vi "Lab8-PSK_Simulation_4PSK_Simple(1).vi"() -> ()   [LabVIEW 2013]
uses:
  <vilib>/addons/Modulation/Digital/General/MT Generate Bits (Galois, PN Order).vi
  <vilib>/addons/Modulation/Digital/General/MT Generate PSK System Parameters(M).vi
  <vilib>/addons/Modulation/Digital/General/MT Generate PSK Synchronization Parameters (bit array).vi
  <vilib>/addons/Modulation/Digital/General/MT Format Eye Diagram (complex).vi
  <vilib>/addons/Modulation/niDMT.lvlib
panel:
  out "sync found index (symbols)":dbl format="%.4f"
  in  "Eb/N0 (dB)":dbl(slide)=48.26086956521739 scale=-10.0..50.0
  out "measurements":T1 caption="Measurements" {"phase offset (deg)" format="%.2f"; "frequency drift (Hz)" format="%.2f"; "frequency offset (Hz)" format="%.2f"}
  out "Baseband Waveform":cluster{"t0":dbl, "dt":dbl, "Y":dbl[]}(graph)
  in  "Tab Control":enum32{"Constellation", "Eye Diagram"}(tab)
  out "Constellation Plot":T2(graph)=[{"constellation"=[-0.6843393450045908, -0.7188173867833647, -0.6862679721424542, -0.7297030487459608, -0.7159912856499204, 0.7221248350001428, -0.69319374455267, -0.7177933374862676, 0.6893145049073991, 0.7164949508669772, -0.7136233597527977, 0.7088022813066004, 0.7026806753460019, 0.6993908820448104, 0.7033303803758204, 0.7023239283689477, -0.7092821972958672, 0.7043694263023035, -0.71123073342578, -0.7063013580615412, 0.7025174893431778, -0.7079249457114573, 0.7056952690720733, -0.711060440916994, -0.7135916049305011, -0.7042966683375681, -0.7053639500078486, -0.7170793110386893, 0.7007122470722706, -0.7041907238690962, 0.7069307076270948, -0.7303032352912369, 0.7036742608538313, -0.7213763894899665, 0.6974920430188264, -0.6906276182534745, 0.7110338385529501, 0.707668395707459, 0.7066450908567875, 0.7156573983712801, 0.7058430026446071, 0.7226424194495579, -0.6941394170921843, 0.7153952742388731, -0.7061754291757949, 0.6989077999376425, 0.7322949703863137, -0.7277124364880128, 0.7152053555332901, -0.7144386806873485, 0.7122523333502172, -0.6946532350705298, -0.6977995339788963], "oversampled data"=[-0.6885507056398621, -0.6904021301332153, -0.701720009748651, 0.7230147663617461, 0.6792985003415442, 0.714980330495899, 0.7083798924531897, -0.7030264642885489, 0.7016069656212314, -0.6995735246622811, -0.7187083014951974, 0.718556461974981, -0.7154964369422703, -0.7143626925937305, -0.7168215682367294, 0.6901290658424636, 0.7193430662186729, 0.7021618219264352, -0.7044915371643418, 0.7010427354068245, 0.72862911894502, -0.6931780204687834, -0.7208414620302925, 0.6898461638663613, 0.7171050214665211, 0.7071101521691305, -0.7158811583840712, 0.7100771986297291, 0.7055043383295747, 0.7197934468495215, -0.7126751015343431, 0.699715799910657, 0.7071055136917425, 0.7000396806158872, 0.6959369636505729, 0.7171363071737368, 0.7097950846368283, 0.707670861017943, 0.6989567675175453, -0.7157042609479739, 0.7040676123623458, 0.7131191099779645, 0.7010491472655718, 0.7001052143691281, -0.7044803945850813, 0.6953086657664377, 0.7183481414573912, 0.7015721146800344, -0.6848840235343148, -0.712341720231345, 0.7005395668208682, 0.6964886799304421, 0.6911618122252481]}, {"constellation"=array[848 elements], "oversampled data"=array[848 elements]}]
  out "Eye Diagram":cluster{"t0":dbl, "dt":dbl, "Y":dbl[]}[](graph)
  in  "M-PSK (4)":i32=4
  out "LED Array":T3
  in  "Message Bits":i32=100
  out "error out":errorcluster
  in  "stop 2":bool
  # "M-PSK Simulation"
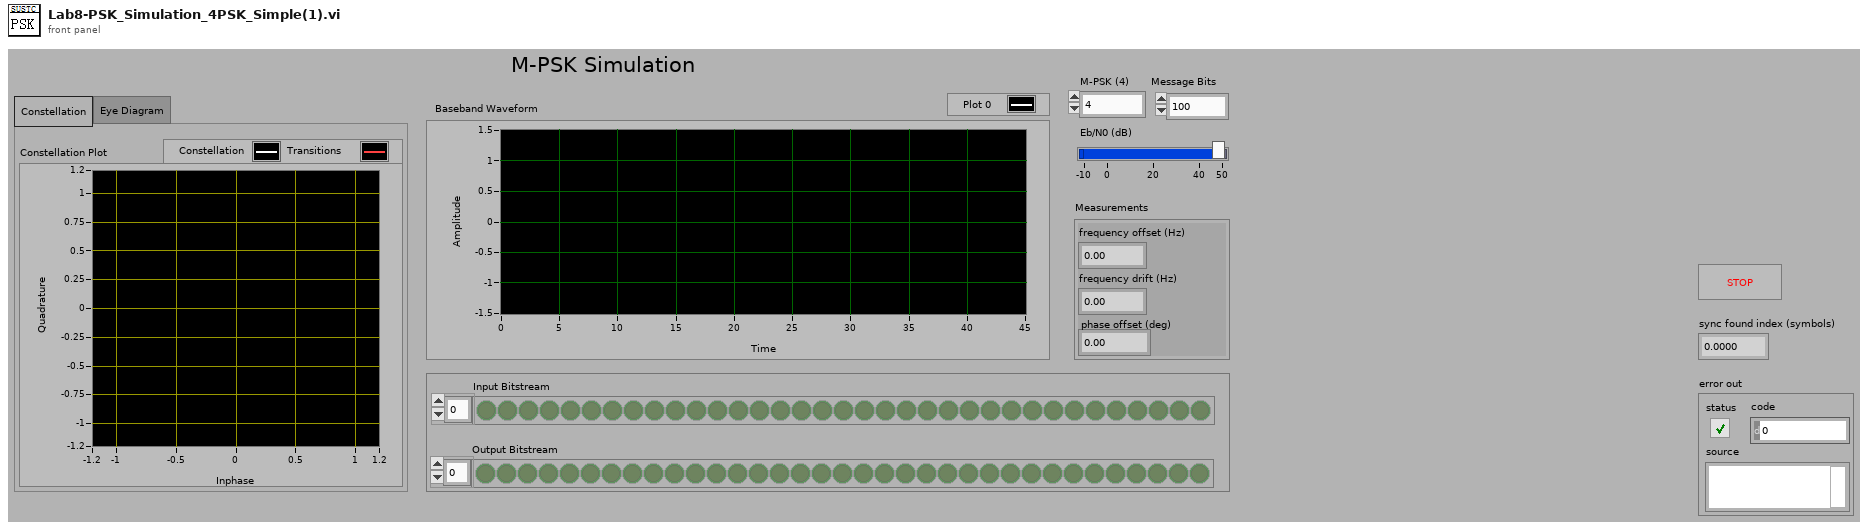
[diagram p1: front panel]
types:
  T1 = cluster{"frequency offset (Hz)":dbl, "frequency drift (Hz)":dbl, "phase offset (deg)":dbl}
  T2 = cluster{"constellation":dbl[], "oversampled data":dbl[]}[]
  T3 = cluster{"Input Bitstream":bool[], "Output Bitstream":bool[]}
  T4 = enum16{"none", "Raised Cosine", "Root Raised Cos", "Gaussian"}
  T5 = enum16{"FSK", "PSK", "QAM", "MSK", "PAM", "ASK", "CPM"}
  T6 = cluster{"samples per symbol (16)":i32, "symbol map":cdb[], "differential PSK":enum16{"disable", "enable"}, "PSK type":u16}
  T7 = typedef "niAMT.lvlib/Complex Data Waveform.ctl" = cluster{"t0":dbl, "dt":dbl, "Y":cdb[]}
  T8 = cluster{"expected sync location (symbols)":i32, "sync sequence":cdb[], "sync location uncertainty (symbols)":i32, "sync indent (symbols)":i32}
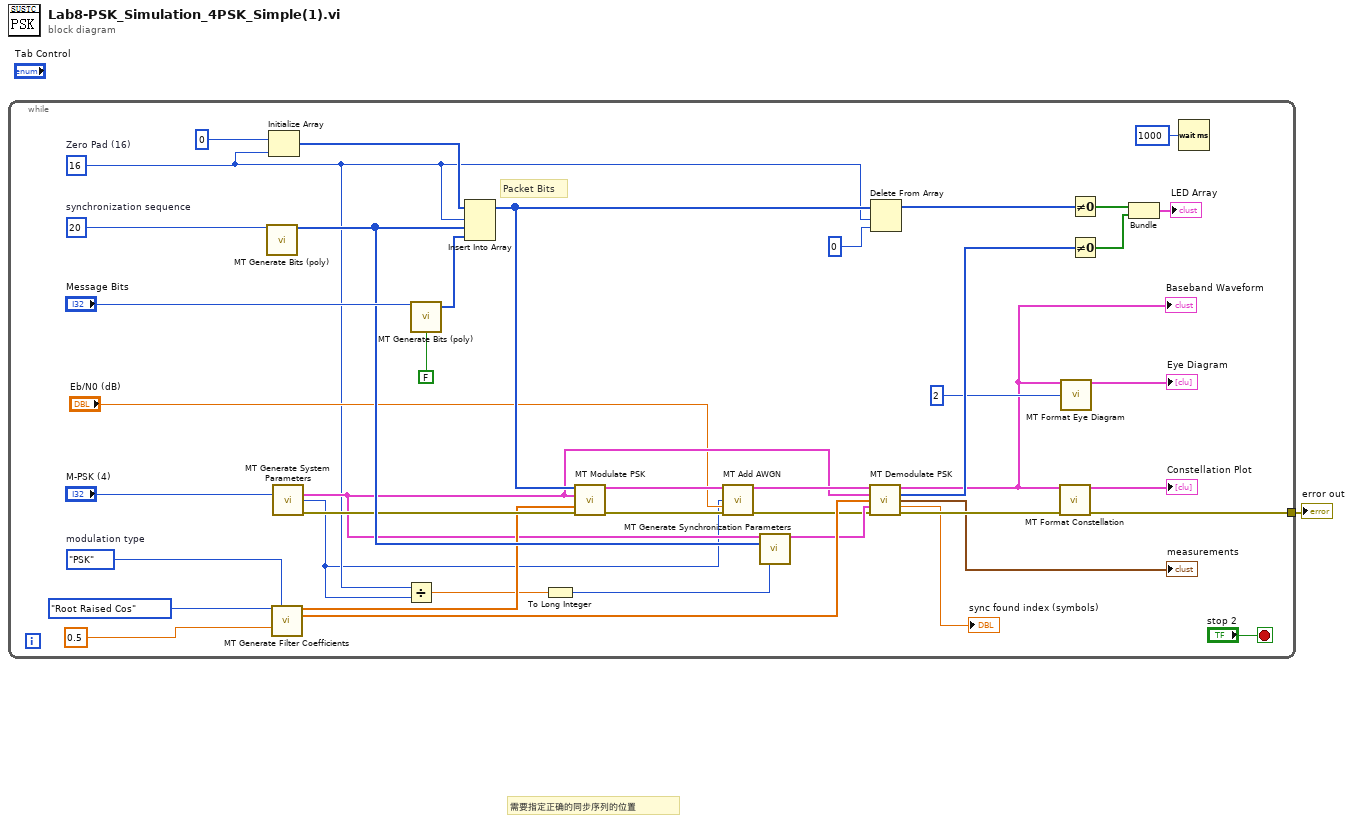
[diagram p0: block diagram]
diagram:
  # "需要指定正确的同步序列的位置"
  n1 = while {
    tunnel: [w22] -> w1
    stop <- "stop 2" stop-if-true
    w5 = 16  # Zero Pad (16)
    w34 = 20  # synchronization sequence
    w43 = T5."PSK"  # modulation type
    # "Packet Bits"
    n2 = call-poly <vilib>:"MT Generate Bits (poly).vi"("total bits (128)"=w34) -> ("output bit stream"=w29:i8[])  [unwired: 12 in, 2 out]
    n3 = Initialize Array(i8 0 ("element"), w5) -> (w26:i8[])
    n4 = call <vilib>:"MT Generate Filter Coefficients.vi"("pulse shaping filter (none)"=T4."Root Raised Cos", "modulation type"=w43, "filter parameter"=0.5) -> ("pulse shaping filter coefficients"=w14:dbl[], "matched filter coefficients"=w35:dbl[])  [unwired: 10 in, 1 out]
    n5 = call-poly <vilib>:"MT Generate System Parameters.vi"("M-PSK (4)"="M-PSK (4)") -> ("PSK system parameters"=w10:T6, "bits per symbol"=w2:i32, "error out"=w24:errorcluster)  [unwired: 12 in]
    n6 = Divide(x=w5, y=w2) -> (x/y=w4:dbl)
    n7 = call-poly <vilib>:"MT Generate Bits (poly).vi"("total bits (128)"="Message Bits", "reset? (T)"=FALSE) -> ("output bit stream"=w30:i8[])  [unwired: 11 in, 2 out]
    n8 = Insert Into Array(array=w26, index=w5, new element #1=w29, new element #2=w30) -> (w33:i8[])
    n9 = To Long Integer(number=w4) -> (32bit integer=w3:i32)
    n10 = call <vilib>:"MT Modulate PSK.vi"("input bit stream"=w33, "PSK system parameters"=w10, "pulse shaping filter coefficients"=w14, "error in (no error)"=w24) -> ("output complex waveform"=w13:T7, "error out"=w8:errorcluster)  [unwired: 9 in, 1 out]
    n11 = call <vilib>:"MT Add AWGN.vi"("input complex waveform"=w13, "bits per symbol (1)"=w2, "Eb/N0 (10 dB)"="Eb/N0 (dB)", "error in (no error)"=w8) -> ("output complex waveform"=w12:T7, "error out"=w9:errorcluster)  [unwired: 9 in, 1 out]
    n12 = call-poly <vilib>:"MT Generate Synchronization Parameters.vi"("PSK system parameters"=w10, "sync bits"=w29, "expected sync location (symbols)"=w3) -> ("PSK synchronization parameters"=w28:T8)  [unwired: 11 in, 1 out]
    n13 = call <vilib>:"MT Demodulate PSK.vi"("input complex waveform"=w12, "PSK system parameters"=w10, "matched filter coefficients"=w35, "synchronization parameters"=w28, "error in (no error)"=w9) -> ("recovered complex waveform"=w18:T7, "output bit stream"=w38:i8[], "measurements"=→"measurements":T1, "sync found index (symbols)"=→"sync found index (symbols)":dbl, "error out"=w23:errorcluster)  [unwired: 6 in]
    "Baseband Waveform" <- w18
    n14 = Delete From Array(array=w33, length=w5, index=0) -> (array with subset deleted=w31:i8[])  [unwired: 1 out]
    n15 = call <vilib>:"MT Format Constellation.vi"("waveform"=w18, "error in (no error)"=w23) -> ("constellation graph"=→"Constellation Plot":T2, "error out"=w22:errorcluster)  [unwired: 12 in]
    n16 = call-poly <vilib>:"MT Format Eye Diagram.vi"("waveform"=w18, "eye length"=2) -> ("eye diagram"=→"Eye Diagram":cluster{"t0":dbl, "dt":dbl, "Y":dbl[]}[])  [unwired: 12 in, 1 out]
    n17 = Not Equal To 0?(x=w31) -> (x != 0?=w41:bool[])
    n18 = Not Equal To 0?(x=w38) -> (x != 0?=w40:bool[])
    n19 = Bundle(w41, w40) -> (→"LED Array":cluster{bool[], bool[]})  [unwired: 1 in]
    n20 = Wait (ms)(milliseconds to wait=u32 1000) -> ()  [unwired: 1 out]
  }
  "error out" <- w1
